vi "BIN_4bit_decimation.vi"(0 "BINARY":string[](array[string])) -> (4 "Final String":string, 5 "10":string, 6 "1":string, 7 "8":string, 8 "2":string, 9 "7":string, 10 "3":string, 11 "9":string, 12 "6":string, 13 "5":string, 14 "4":string, 15 "Array":string[](array[string]))   [LabVIEW 2021]
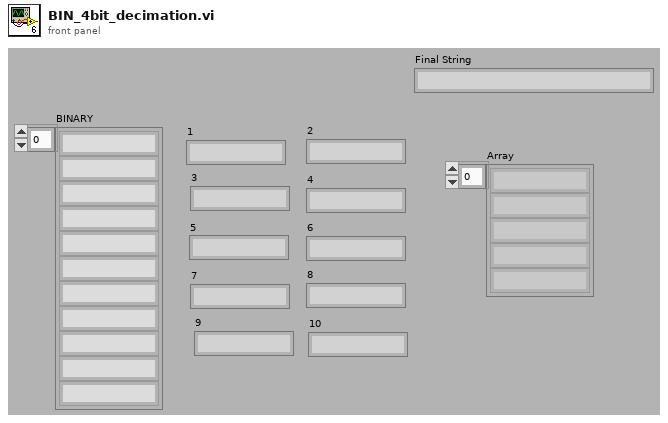
[diagram p1: front panel]
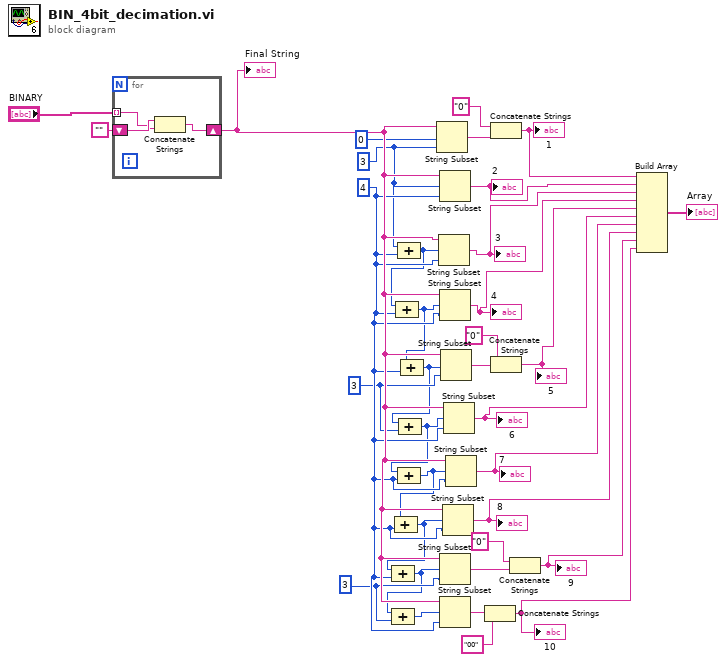
[diagram p0: block diagram]
diagram:
  w18 = 3 ("length (rest)")
  w10 = 3 ("length (rest)")
  w19 = 4 ("length (rest)")
  w4 = 3 ("length (rest)")
  n1 = for {
    tunnel: "BINARY" -> [w36] mode=indexing
    shift-right: [w38] -> w35
    shift-left: "" -> [w37]
    n2 = Concatenate Strings(w37, w36) -> (w38:string)
  }
  "Final String" <- w35
  n3 = Compound Arithmetic op=unknown(w4, w19) -> (w5:i32)
  n4 = Compound Arithmetic op=unknown(w5, w19) -> (w7:i32)
  n5 = Compound Arithmetic op=unknown(w7, w19) -> (w9:i32)
  n6 = Compound Arithmetic op=unknown(w9, w10) -> (w11:i32)
  n7 = Compound Arithmetic op=unknown(w11, w19) -> (w12:i32)
  n8 = Compound Arithmetic op=unknown(w12, w19) -> (w13:i32)
  n9 = Compound Arithmetic op=unknown(w13, w19) -> (w17:i32)
  n10 = Compound Arithmetic op=unknown(w17, w18) -> (w16:i32)
  n11 = String Subset(string=w35, offset (0)=0, length (rest)=w4) -> (substring=w3:string)
  n12 = String Subset(string=w35, offset (0)=w5, length (rest)=w19) -> (substring=w24:string)
  "3" <- w24
  n13 = String Subset(string=w35, offset (0)=w4, length (rest)=w19) -> (substring=w23:string)
  "2" <- w23
  n14 = String Subset(string=w35, offset (0)=w7, length (rest)=w19) -> (substring=w25:string)
  "4" <- w25
  n15 = String Subset(string=w35, offset (0)=w17, length (rest)=w18) -> (substring=w15:string)
  n16 = String Subset(string=w35, offset (0)=w16, length (rest)=w19) -> (substring=w20:string)
  n17 = String Subset(string=w35, offset (0)=w9, length (rest)=w10) -> (substring=w8:string)
  n18 = String Subset(string=w35, offset (0)=w13, length (rest)=w19) -> (substring=w29:string)
  "8" <- w29
  n19 = String Subset(string=w35, offset (0)=w11, length (rest)=w19) -> (substring=w27:string)
  "6" <- w27
  n20 = String Subset(string=w35, offset (0)=w12, length (rest)=w19) -> (substring=w28:string)
  "7" <- w28
  n21 = Concatenate Strings(w20, "00" ("string")) -> (w31:string)
  "10" <- w31
  n22 = Concatenate Strings("0" ("string"), w3) -> (w22:string)
  "1" <- w22
  n23 = Concatenate Strings("0" ("string"), w8) -> (w26:string)
  "5" <- w26
  n24 = Concatenate Strings("0" ("string"), w15) -> (w30:string)
  "9" <- w30
  n25 = Build Array(w22, w23, w24, w25, w26, w27, w28, w29, w30, w31) -> (→"Array":string[])
